vi "Tellop Drive Code.vi"(4 "Buttons":T22, 6 "Axes":T23, 8 "error in (no error)":errorcluster, 9 "Shifter from Shift":T24, 10 "Manual?":bool, 11 "Drive":T1) -> (0 "error out":errorcluster, 1 "Shifter to Shift":T24, 2 "Robot speed in FPS":dbl, 3 "Drive out":T1, 5 "in High Gear?":bool, 7 "Recomended Gear (may be in that gear)":bool)   [LabVIEW 2013]
uses:
  Drive typedef.ctl
  Drive Motors Typedef.ctl
  GearBox Typedef.ctl
  <vilib>/Rock Robotics/WPI/MotorControl/WPI_MotorControlDeviceRef.ctl
  <vilib>/Rock Robotics/SystemInterfaces/Typedef/FPGA_TypedefDigitalModule.ctl
  <vilib>/Rock Robotics/SystemInterfaces/DIO/FPGA_DIOPWMChannel.ctl
  <vilib>/Rock Robotics/WPI/PWM/WPI_PWMDeadband.ctl
  <vilib>/Rock Robotics/WPI/CAN/Jaguar/SubVIs/WPI_CANJaguar_ControlMode.ctl
  <vilib>/Rock Robotics/WPI/PWM/WPI_PWMTransform_ConPane.ctl
  <vilib>/Rock Robotics/WPI/Solenoid/WPI_SolenoidDevRef.ctl
  <vilib>/Rock Robotics/SystemInterfaces/Typedef/FPGA_TypedefSolenoidModule.ctl
  <vilib>/Rock Robotics/WPI/Solenoid/WPI_SolenoidChannel.ctl
  Drive Sensor Typedef.ctl
  <vilib>/Rock Robotics/WPI/Encoder/WPI_EncoderDevRef.ctl
  <vilib>/Rock Robotics/SystemInterfaces/Encoder/FPGA_EncoderIdx.ctl
  <vilib>/Rock Robotics/SystemInterfaces/Counter/FPGA_CounterCtrSystemIndex.ctl
  <vilib>/Rock Robotics/WPI/Encoder/WPI_EncoderType.ctl
  <vilib>/Rock Robotics/WPI/Gyro/WPI_GyroDevRef.ctl
  <vilib>/Rock Robotics/SystemInterfaces/Typedef/FPGA_TypedefAnalogModule.ctl
  <vilib>/Rock Robotics/SystemInterfaces/AI/FPGA_AIChannel.ctl
  Auto Transmission Code/All Shifter shift register typedef.ctl
  Auto Transmission Code/Shifter shift typedef.ctl
  <vilib>/Rock Robotics/WPI/Joystick/WPI_JoystickButtonState.ctl
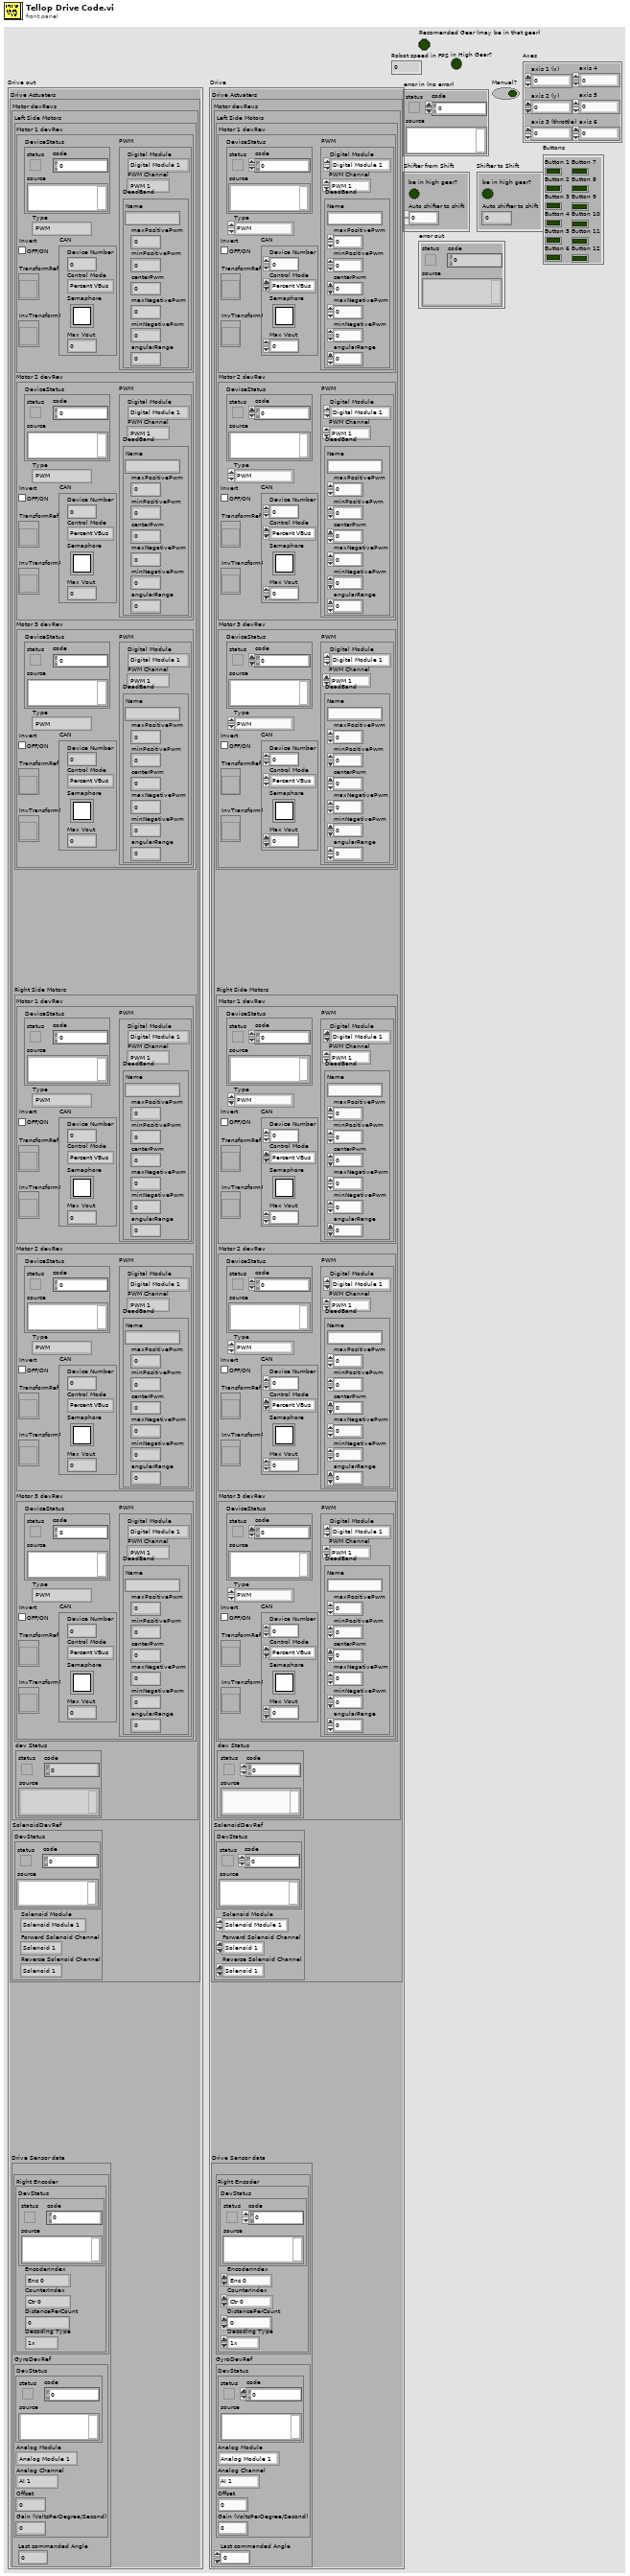
[diagram p1: front panel]
types:
  T1 = typedef "Drive typedef.ctl" = cluster{"Drive Actuaters":cluster{"Motor devRevs":T2, "SolenoidDevRef":T11}, "Drive Sensor data":T14}
  T2 = typedef "Drive Motors Typedef.ctl" = cluster{"Left Side Motors":T3, "Right Side Motors":T3, "dev Status":errorcluster}
  T3 = typedef "GearBox Typedef.ctl" = cluster{"Motor 1 devRev":T4, "Motor 2 devRev":T4, "Motor 3 devRev":T4}
  T4 = typedef "WPI_MotorControlDeviceRef.ctl" = cluster{"DeviceStatus":errorcluster, "Type":enum16{"PWM", "CAN"}, "PWM":cluster{"Digital Module":T5, "PWM Channel":T6, "DeadBand":T7}, "CAN":cluster{"Device Number":u8, "Control Mode":T8, "Semaphore":T9, "Max Vout":dbl}, "Invert":bool, "TransformRef":T10, "InvTransformRef":T10}
  T5 = typedef "FPGA_TypedefDigitalModule.ctl" = enum16{"Digital Module 1", "Digital Module 2"}
  T6 = typedef "FPGA_DIOPWMChannel.ctl" = enum8{"PWM 1", "PWM 2", "PWM 3", "PWM 4", "PWM 5", "PWM 6", "PWM 7", "PWM 8", "PWM 9", "PWM 10", "Invalid"}
  T7 = typedef "WPI_PWMDeadband.ctl" = cluster{"Name":string, "maxPositivePwm":i32, "minPositivePwm":i32, "centerPwm":i32, "maxNegativePwm":i32, "minNegativePwm":i32, "angularRange":u16}
  T8 = typedef "WPI_CANJaguar_ControlMode.ctl" = enum8{"Percent VBus", "Current", "Speed", "Position", "Voltage"}
  T9 = typedef "Semaphore RefNum" = refnum<k1>
  T10 = typedef "WPI_PWMTransform_ConPane.ctl" = refnum<vi>
  T11 = typedef "WPI_SolenoidDevRef.ctl" = cluster{"DevStatus":errorcluster, "Solenoid Module":T12, "Forward Solenoid Channel":T13, "Reverse Solenoid Channel":T13}
  T12 = typedef "FPGA_TypedefSolenoidModule.ctl" = enum16{"Solenoid Module 1", "Solenoid Module 2"}
  T13 = typedef "WPI_SolenoidChannel.ctl" = enum8{"Solenoid 1", "Solenoid 2", "Solenoid 3", "Solenoid 4", "Solenoid 5", "Solenoid 6", "Solenoid 7", "Solenoid 8", "Invalid"}
  T14 = typedef "Drive Sensor Typedef.ctl" = cluster{"Encoders":cluster{"Right Encoder":T15}, "GyroDevRef":T19, "Last commanded Angle":dbl}
  T15 = typedef "WPI_EncoderDevRef.ctl" = cluster{"DevStatus":errorcluster, "EncoderIndex":T16, "CounterIndex":T17, "DistancePerCount":dbl, "Decoding Type":T18}
  T16 = typedef "FPGA_EncoderIdx.ctl" = enum8{"Enc 0", "Enc 1", "Enc 2", "Enc 3", "Invalid"}
  T17 = typedef "FPGA_CounterCtrSystemIndex.ctl" = enum8{"Ctr 0", "Ctr 1", "Ctr 2", "Ctr 3", "Ctr 4", "Ctr 5", "Ctr 6", "Ctr 7", "Invalid"}
  T18 = typedef "WPI_EncoderType.ctl" = enum16{"1x", "2x", "4x"}
  T19 = typedef "WPI_GyroDevRef.ctl" = cluster{"DevStatus":errorcluster, "Analog Module":T20, "Analog Channel":T21, "Offset":dbl, "Gain (VoltsPerDegree/Second)":dbl}
  T20 = typedef "FPGA_TypedefAnalogModule.ctl" = enum16{"Analog Module 1", "Analog Module 2"}
  T21 = typedef "FPGA_AIChannel.ctl" = enum8{"AI 1", "AI 2", "AI 3", "AI 4", "AI 5", "AI 6", "AI 7", "AI 8", "Invalid"}
  T22 = typedef "WPI_JoystickButtonState.ctl" = cluster{"Button 1":bool, "Button 2":bool, "Button 3":bool, "Button 4":bool, "Button 5":bool, "Button 6":bool, "Button 7":bool, "Button 8":bool, "Button 9":bool, "Button 10":bool, "Button 11":bool, "Button 12":bool}
  T23 = cluster{"axis 1 (x)":dbl, "axis 2 (y)":dbl, "axis 3 (throttle)":dbl, "axis 4":dbl, "axis 5":dbl, "axis 6":dbl}
  T24 = typedef "All Shifter shift register typedef.ctl" = cluster{"be in high gear?":bool, "Auto shifter to shift":T25}
  T25 = typedef "Shifter shift typedef.ctl" = u32
  T26 = typedef "All Shifter Constants.ctl" = cluster{"Drive info constants":cluster{"Enocder Pulses per foot":dbl, "Amount of turn before drive is turning":dbl}, "Shift control Constants":T27}
  T27 = typedef "Shift Constants.ctl" = cluster{"Global shift constants":cluster{"Mili seconds before it can shift again":u32, "Max fps":dbl}, "Upshift constants":cluster{"Upshift point in fps":dbl, "Upshift Accel constant":dbl, "Commanded Throttle  shiftpoint gain":dbl}, "Downshift Constants":cluster{"Kickdown shift point":dbl, "Kickdown at -acceleration":dbl, "Slowest Throttle for kickdown":dbl, "Coastdown shift speed":dbl}}
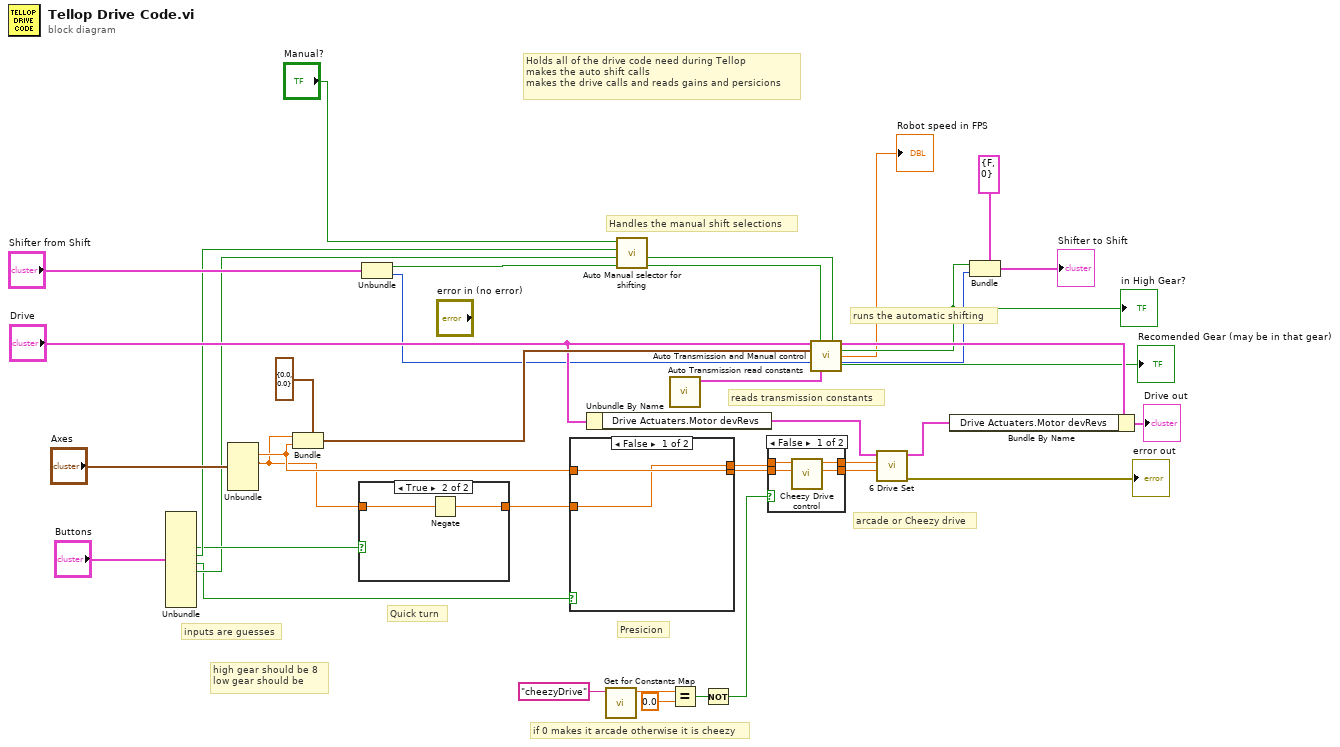
[diagram p0: block diagram]
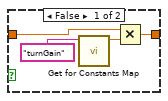
[diagram p2: hidden frame]
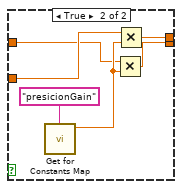
[diagram p3: hidden frame]
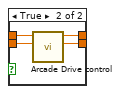
[diagram p4: hidden frame]
diagram:
  # "high gear should be 8\nlow gear should be"
  # "runs the automatic shifting"
  # "reads transmission constants"
  # "if 0 makes it arcade otherwise it is cheezy"
  # "Handles the manual shift selections"
  # "Holds all of the drive code need during Tellop\nmakes the auto shift calls\nmakes the drive calls and reads gains and persicions"
  # "inputs are guesses"
  # "Presicion"
  # "Quick turn"
  # "arcade or Cheezy drive"
  n1 = Unbundle("Buttons") -> ("Button 5"=w4:bool, "Button 6"=w5:bool, "Button 7"=w2:bool, "Button 8"=w3:bool)  [unwired: 8 out]
  n2 = Unbundle("Axes") -> ("axis 2 (y)"=w26:dbl, "axis 3 (throttle)"=w6:dbl)  [unwired: 4 out]
  n3 = Bundle(cluster=cluster{"Steer":dbl, "Throttle":dbl} {"Steer"=0.0, "Throttle"=0.0} ("Commanded speeds"), "Steer"=w6, "Throttle"=w26) -> (w36:cluster{"Steer":dbl, "Throttle":dbl})
  n4 = case shown="True" w4 {
    tunnel: w6 -> [w43 w45]
    tunnel: [w40 w44] -> w24
    frame False {
      n5 = call "Get for Constants Map.vi"("Constant Name"="turnGain") -> ("Value"=w41:dbl)  [unwired: 8 in, 2 out]
      n6 = Multiply(x=w43, y=w41) -> (x*y=w40:dbl)
    }
    frame True {
      n7 = Negate(x=w45) -> (-x=w44:dbl)
    }
  }
  n8 = Unbundle("Shifter from Shift") -> ("be in high gear?"=w14:bool, "Auto shifter to shift"=w22:T25)
  n9 = case shown="False" w2 {
    tunnel: w26 -> [w47 w48]
    tunnel: w24 -> [w46 w52]
    tunnel: [w47 w51] -> w25
    tunnel: [w46 w53] -> w1
    frame False {
    }
    frame True {
      n10 = call "Get for Constants Map.vi"("Constant Name"="presicionGain") -> ("Value"=w49:dbl)  [unwired: 8 in, 2 out]
      n11 = Multiply(x=w48, y=w49) -> (x*y=w51:dbl)
      n12 = Multiply(x=w52, y=w49) -> (x*y=w53:dbl)
    }
  }
  n13 = Unbundle By Name("Drive") -> ("Drive Actuaters.Motor devRevs"=w34:T2)
  n14 = call "Get for Constants Map.vi"("Constant Name"="cheezyDrive") -> ("Value"=w30:dbl)  [unwired: 8 in, 2 out]
  n15 = call "Auto Manual selector for shifting.vi"("From Shift"=w14, "High Gear button"=w3, "Low Gear button"=w5, "Manual?"="Manual?") -> ("Manually controlled"=w15:bool, "High Gear?"=w16:bool)  [unwired: 6 in]
  n16 = call "Auto Transmission read constants.vi"() -> ("All Shifter Constants"=w31:T26)  [unwired: 10 in, 1 out]
  n17 = Equal?(x=w30, y=0.0) -> (x = y?=w28:bool)
  n18 = Not(x=w28) -> (.not. x?=w7:bool)
  n19 = case shown="False" w7 {
    tunnel: w25 -> [w57 w60]
    tunnel: w1 -> [w56 w61]
    tunnel: [w55 w59] -> w38
    tunnel: [w54 w58] -> w37
    frame False {
      n20 = call "Cheezy Drive control.vi"("Throttle"=w57, "Steer"=w56) -> ("Right motor output"=w54:dbl, "Left motor ouput"=w55:dbl)  [unwired: 8 in]
    }
    frame True {
      n21 = call "Arcade Drive control.vi"("Throttle"=w60, "Steer"=w61) -> ("right side"=w58:dbl, "left side"=w59:dbl)  [unwired: 8 in]
    }
  }
  n22 = call "Auto Transmission and Manual control.vi"("Drive"="Drive", "Force which gear it is in"=w15, "Forced high gear?"=w16, "Commanded speeds"=w36, "from Shift"=w22, "All Shifter Constants"=w31) -> ("Drive out"=w33:T1, "in High Gear?"=w17:bool, "Robot speed in FPS"=→"Robot speed in FPS":dbl, "To shift"=w19:T25, "Recomended Gear (may be in that gear)"=→"Recomended Gear (may be in that gear)":bool)  [unwired: 4 in, 1 out]
  "in High Gear?" <- w17
  n23 = call "6 Drive Set.vi"("Motor devRevs"=w34, "Left side speed"=w38, "Right side speed"=w37) -> ("Motor devRevs"=w32:T2, "error out"=→"error out":errorcluster)  [unwired: 6 in]
  n24 = Bundle By Name(cluster=w33, "Drive Actuaters.Motor devRevs"=w32) -> (→"Drive out":T1)
  n25 = Bundle(cluster=T24 {"be in high gear?"=FALSE, "Auto shifter to shift"=0} ("Shifter to Shift 2"), "be in high gear?"=w17, "Auto shifter to shift"=w19) -> (→"Shifter to Shift":T24)
